vi "fgv_Ref_AVI_Globals.vi"(0 "AVI mode":T1, 2 "Function":enum16{"Intialize", "Write", "Read", "Clear"}(ring), 5 "Red Ref AVI":T2, 7 "Green Ref AVI":T2, 11 "error in (no error)":errorcluster, 13 "\"Write\" sub function":T6(ring)=enum."Write Green AVI") -> (4 "AVI mode":T1, 6 "Red Ref AVI":T2, 8 "Green Ref AVI":T2, 15 "error out":errorcluster)   [LabVIEW 2017]
uses:
  Typedefs/AVI Refs cluster.ctl
  <vilib>/vision/Avi.llb/IMAQ AVI2 Refnum.ctl
  <vilib>/vision/Image Controls.llb/IMAQ Image.ctl
  <vilib>/vision/Avi1.llb/AviRefnum.ctl
  Typedefs/AVI implementation enum.ctl
panel:
  # "SUBROUTINE VI"
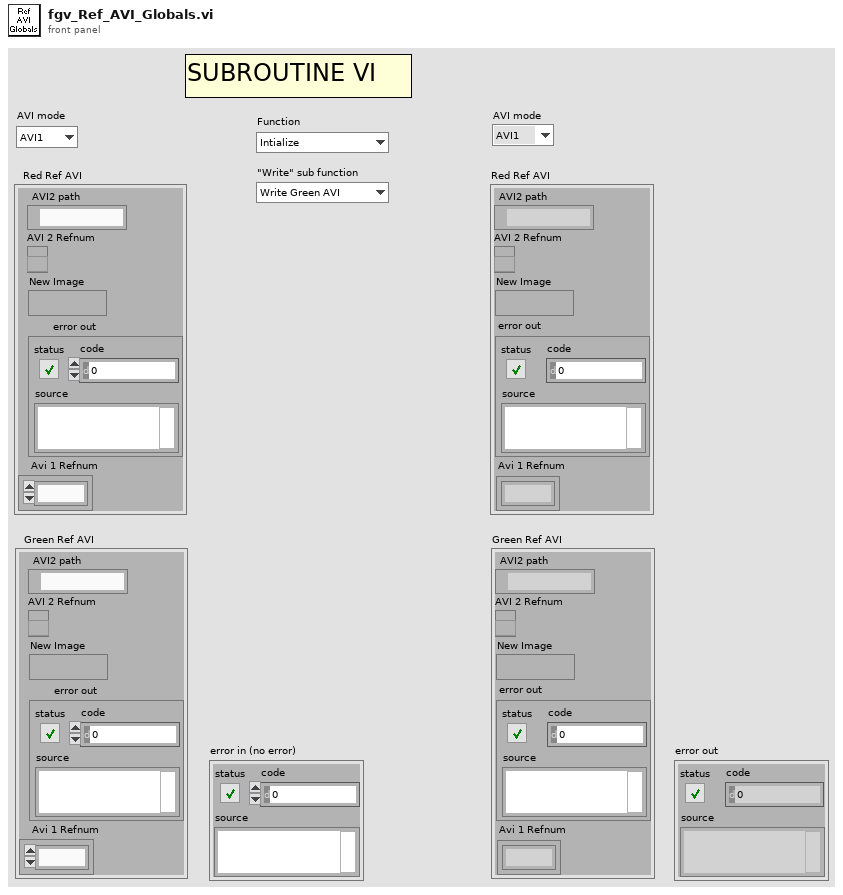
[diagram p1: front panel]
types:
  T1 = typedef "AVI implementation enum.ctl" = enum16{"AVI1", "AVI2"}
  T2 = typedef "AVI Refs cluster.ctl" = cluster{"AVI2 path":path, "AVI 2 Refnum":T3, "New Image":T4, "error out":errorcluster, "Avi 1 Refnum":T5}
  T3 = typedef "IMAQ AVI2 Refnum.ctl" = refnum<k20>
  T4 = typedef "IMAQ Image.ctl" = refnum<image>
  T5 = typedef "AviRefnum.ctl" = refnum<k1>
  T6 = enum16{"Write Red AVI", "Write Green AVI", "Write AVI mode"}
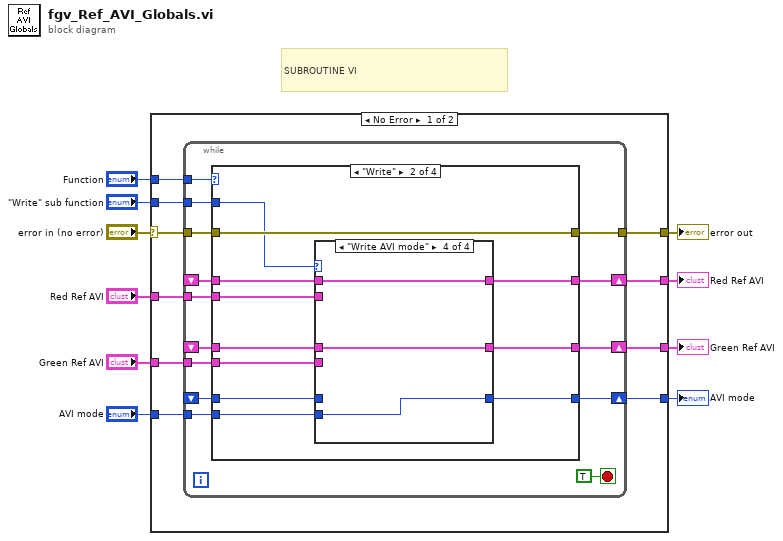
[diagram p0: block diagram]
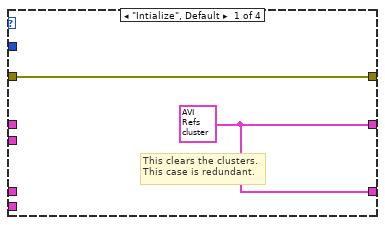
[diagram p2: hidden frame]
diagram:
  # "SUBROUTINE VI"
  n1 = case shown="No Error" "error in (no error)" {
    selector: "error in (no error)" -> [w17 w68]
    tunnel: [w18 w68] -> w9
    tunnel: "Function" -> [w20 _]
    tunnel: "Red Ref AVI" -> [w19 w67]
    tunnel: [w16 w67] -> w7
    tunnel: "Green Ref AVI" -> [w15 w66]
    tunnel: [w14 w66] -> w6
    tunnel: "AVI mode" -> [w13 w65]
    tunnel: "\"Write\" sub function" -> [w12 _]
    tunnel: [w11 w65] -> w1
    frame No Error {
      n2 = while {
        tunnel: w20 -> [w33]
        tunnel: w19 -> [w32]
        shift-right: [w31] -> w16
        shift-left: _ -> [w30]
        tunnel: [w28] -> w18
        tunnel: w17 -> [w29]
        tunnel: w15 -> [w27]
        shift-right: [w26] -> w14
        shift-left: _ -> [w25]
        tunnel: w13 -> [w24]
        shift-right: [w23] -> w11
        shift-left: _ -> [w22]
        tunnel: w12 -> [w21]
        stop <- TRUE stop-if-true
        n3 = case shown="\"Write\"" w33 {
          tunnel: [w35 w41 w63 _] -> w31
          tunnel: w32 -> [_ w45 _ _]
          tunnel: w30 -> [_ w40 w63 _]
          tunnel: [w36 w47 w62 w64] -> w28
          tunnel: w29 -> [w36 w47 w62 w64]
          tunnel: w27 -> [_ w46 _ _]
          tunnel: [w35 w39 w61 _] -> w26
          tunnel: w25 -> [_ w42 w61 _]
          tunnel: w24 -> [_ w44 _ _]
          tunnel: [_ w37 w60 _] -> w23
          tunnel: w22 -> [_ w38 w60 _]
          tunnel: w21 -> [_ w43 _ _]
          frame "Intialize", Default {
            w35 = T2 {"AVI2 path"=path "", "AVI 2 Refnum"=refnum, "New Image"=refnum, "error out"={"status"=FALSE, "code"=0, "source"=""}, "Avi 1 Refnum"=refnum} ("Red AVI")
            # "This clears the clusters.\nThis case is redundant."
          }
          frame "Write" {
            n4 = case shown="\"Write AVI mode\"" w43 {
              tunnel: w46 -> [_ _ w56 _]
              tunnel: w45 -> [_ w52 _ _]
              tunnel: w44 -> [_ _ _ w57]
              tunnel: w42 -> [w49 w53 _ w58]
              tunnel: [w50 w52 w55 w59] -> w41
              tunnel: w40 -> [w50 _ w55 w59]
              tunnel: [w49 w53 w56 w58] -> w39
              tunnel: [w48 w51 w54 w57] -> w37
              tunnel: w38 -> [w48 w51 w54 _]
              frame Default {
              }
              frame "Write Red AVI" {
              }
              frame "Write Green AVI" {
              }
              frame "Write AVI mode" {
              }
            }
          }
          frame "Read" {
          }
          frame "Clear" {
          }
        }
      }
    }
    frame Error {
    }
  }
  "error out" <- w9
  "Red Ref AVI" <- w7
  "Green Ref AVI" <- w6
  "AVI mode" <- w1
